vi "Test_WriteValue_TransportClosed_Error.vi"(8 "error in (no error)":errorcluster, 11 "TestCase in":refnum<class "TestValueReferenceTransport.lvclass">) -> (0 "error out":errorcluster, 3 "TestCase out":refnum<class "TestValueReferenceTransport.lvclass">)   [LabVIEW 2017, in "TestValueReferenceTransport.lvclass"]
uses:
  TestValueReferenceTransport.lvclass
  Source/Concrete/ValueReferenceTransport/ValueReferenceTransport.lvclass
  C:/Git/composed-transport/Source/ITransport/ITransport.lvclass
  Source/ITransport/ITransport.lvclass
panel:
  out "Return Error":errorcluster
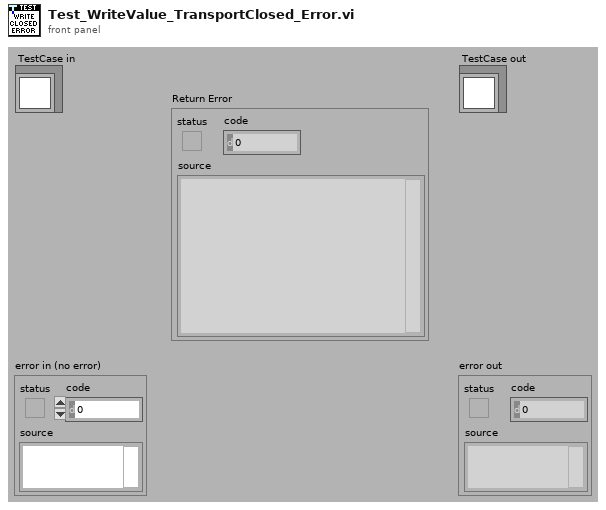
[diagram p1: front panel]
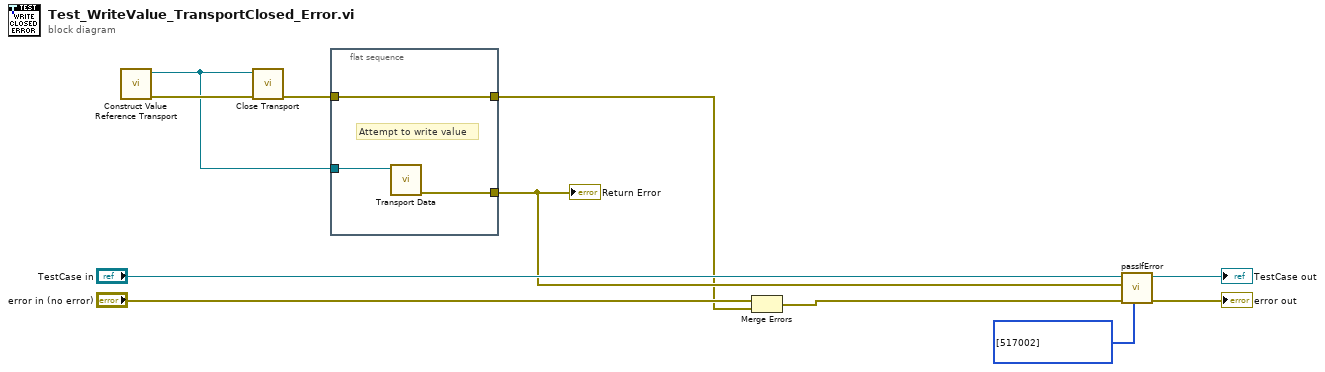
[diagram p0: block diagram]
diagram:
  n1 = call "Construct Value Reference Transport.vi"() -> ("error out"=w5:errorcluster, "ValueReferenceTransport"=w3:refnum<class "ValueReferenceTransport.lvclass">)  [unwired: 10 in]
  n2 = call-dynamic "Close Transport.vi"("error in (no error)"=w5, "ValueReferenceTransport in"=w3) -> ("error out"=w2:errorcluster)  [unwired: 9 in]
  n3 = flat-sequence {
    tunnel: [w14] -> w4
    tunnel: w3 -> [w13]
    tunnel: w2 -> [w12]
    tunnel: [w12] -> w1
    frame #0 {
      # "Attempt to write value"
      n4 = call "Transport Data.vi"("ITransport in"=w13) -> ("error out"=w14:errorcluster)  [unwired: 9 in, 1 out]
    }
  }
  n5 = Merge Errors("error in (no error)", w1) -> (w6:errorcluster)
  n6 = call-dynamic "passIfError.vi"("passing error codes (default = any error code)"=i32[] [517002], "error in (no error)"=w6, "error"=w4, "TestCase in"="TestCase in") -> ("error out"=→"error out":errorcluster, "TestCase out"=→"TestCase out":refnum<class "TestValueReferenceTransport.lvclass">)  [unwired: 6 in]
  "Return Error" <- w4
